vi "ProdaNG.Product.Get.vi"(8 "error in (no error)":errorcluster, 9 "serialNumber":string, 10 "wabcoPartId":i32, 11 "dbHandle":i32) -> (0 "error out":errorcluster, 1 "found":bool, 2 "Product":T1, 3 "dbHandle out":i32)   [LabVIEW 2016]
doc: "This function returns a product structure for a product, which is identified by a part and a serial number.\nImportant information: The field 'individual' was taken over from the field 'allgemein' of the legacy data directly. Because of this most products have the value 0 further on and only a few the value 1. \nParameter:\nhandle is an Integer, which is returned by the function Login() at the creation of a new connection.\nwabcoPartId is the Id of the part.\nserialNumber is the serial number of the product for the part above.\nproduct is a pointer on a product structure, which is filled if the returncode is 0. The structure must be defined in the calling program.\n\nReturncodes:\n0 No error\n< 0 ORACLE Error code\n6 (ERROR_INVALID_HANDLE) in case of an invalid handle\n1403 Record does not exist"
uses:
  Controls/ProdaNG.Product.ctl
  Controls/ProdaNG.ProductSize.ctl
  prodllNG.dll
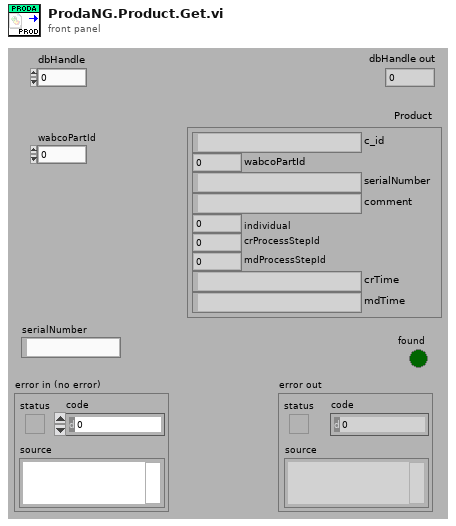
[diagram p1: front panel]
types:
  T1 = typedef "ProdaNG.Product.ctl" = cluster{"c_id":string, "wabcoPartId":i32, "serialNumber":string, "comment":string, "individual":i32, "crProcessStepId":i32, "mdProcessStepId":i32, "crTime":string, "mdTime":string}
  T2 = typedef "ProdaNG.ProductSize.ctl" = cluster{"c_id":i32, "wabcoPartId":i32, "serialNumber":i32, "comment":i32, "individual":i32, "crProcessStepId":i32, "mdProcessStepId":i32, "crTime":i32, "mdTime":i32}
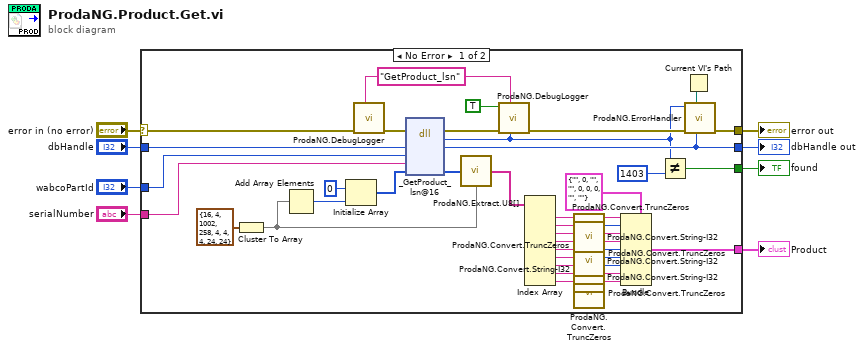
[diagram p0: block diagram]
diagram:
  n1 = case shown="No Error" "error in (no error)" {
    selector: "error in (no error)" -> [w45 w52]
    tunnel: [w50 w52] -> w7
    tunnel: "dbHandle" -> [w47 w51]
    tunnel: [w48 w51] -> w5
    tunnel: "wabcoPartId" -> [w32 _]
    tunnel: "serialNumber" -> [w31 _]
    tunnel: [w19 _] -> w2
    tunnel: [w39 _] -> w1
    frame No Error {
      w41 = "GetProduct_lsn" ("cmd")
      n2 = Cluster To Array(cluster=T2 {"c_id"=16, "wabcoPartId"=4, "serialNumber"=1002, "comment"=258, "individual"=4, "crProcessStepId"=4, "mdProcessStepId"=4, "crTime"=24, "mdTime"=24} ("ProductSize")) -> (array=w34:i32[])
      n3 = Add Array Elements(numeric array=w34) -> (sum=w33:i32)
      n4 = Initialize Array(u8 0 ("element"), w33) -> (w37:u8[])
      n5 = call "ProdaNG.DebugLogger.vi"("cmd"=w41, "error in (no error)"=w45) -> ("error out"=w44:errorcluster)  [unwired: 9 in]
      n6 = dll-call lib="D:/Maszup/WABCO/SVN/LineTraceSystem/SOFTWARE/sources/Database/ProdaNG/prodllNG.dll" fn="_GetProduct_lsn@16" ("ProDLL wrapper.dll:ProDLL_wrapper_GetWabcoParts_GetData")(error in=w44, "dbHandle"=w47, "wabcoProductId"=w32, "serialNumber"=w31, "product"=w37) -> (error out=w43:errorcluster, "return type"=w21:i32, "dbHandle"=w48:i32, "product"=w35:u8[])  [unwired: 4 in, 1 out]
      n7 = call "ProdaNG.Extract.U8[].vi"("unsigned byte array"=w35, "Sizes"=w34) -> ("Elements"=w30:string[])
      n8 = call "ProdaNG.DebugLogger.vi"("return type"=w21, "cmd"=w41, "error in (no error)"=w43, "done? (F)"=TRUE) -> ("error out"=w42:errorcluster)  [unwired: 7 in]
      n9 = Index Array(array=w30) -> (element #1=w10:string, element #2=w28:string, element #3=w18:string, element #4=w17:string, element #5=w27:string, element #6=w25:string, element #7=w23:string, element #8=w14:string, element #9=w13:string)  [unwired: 9 in]
      n10 = call "ProdaNG.Convert.TruncZeros.vi"("string with \\0s"=w10) -> ("LV string"=w9:string)  [unwired: 10 in]
      n11 = call "ProdaNG.Convert.String-I32.vi"("unsigned byte string"=w28) -> ("32bit integer"=w29:i32)  [unwired: 10 in]
      n12 = call "ProdaNG.Convert.TruncZeros.vi"("string with \\0s"=w18) -> ("LV string"=w16:string)  [unwired: 10 in]
      n13 = call "ProdaNG.Convert.TruncZeros.vi"("string with \\0s"=w17) -> ("LV string"=w15:string)  [unwired: 10 in]
      n14 = call "ProdaNG.Convert.String-I32.vi"("unsigned byte string"=w27) -> ("32bit integer"=w26:i32)  [unwired: 10 in]
      n15 = call "ProdaNG.Convert.String-I32.vi"("unsigned byte string"=w25) -> ("32bit integer"=w24:i32)  [unwired: 10 in]
      n16 = call "ProdaNG.Convert.String-I32.vi"("unsigned byte string"=w23) -> ("32bit integer"=w22:i32)  [unwired: 10 in]
      n17 = call "ProdaNG.Convert.TruncZeros.vi"("string with \\0s"=w14) -> ("LV string"=w12:string)  [unwired: 10 in]
      n18 = call "ProdaNG.Convert.TruncZeros.vi"("string with \\0s"=w13) -> ("LV string"=w11:string)  [unwired: 10 in]
      n19 = Bundle(cluster=T1 {"c_id"="", "wabcoPartId"=0, "serialNumber"="", "comment"="", "individual"=0, "crProcessStepId"=0, "mdProcessStepId"=0, "crTime"="", "mdTime"=""} ("Product"), "c_id"=w9, "wabcoPartId"=w29, "serialNumber"=w16, "comment"=w15, "individual"=w26, "crProcessStepId"=w24, "mdProcessStepId"=w22, "crTime"=w12, "mdTime"=w11) -> (w39:T1)
      n20 = Not Equal?(x=w21, y=1403) -> (x != y?=w19:bool)
      n21 = Current VI's Path() -> (path=w49:path)
      n22 = call "ProdaNG.ErrorHandler.vi"("dbHandleIn"=w48, "Path"=w49, "error in"=w42, "output_parameter"=w21) -> ("error out"=w50:errorcluster)  [unwired: 7 in]
    }
    frame Error {
    }
  }
  "error out" <- w7
  "dbHandle out" <- w5
  "found" <- w2
  "Product" <- w1
